vi "Get Profile Extract Cnt.vi"(8 "Profile Cnt (0: rest)":u32, 9 "Profile Index (0)":u32, 10 "Profile Info":T1, 11 "Profile Data":u32[](array[numeric])) -> (3 "Extract Cnt":u32)   [LabVIEW 2014, in "Keyence LJ-V7000.lvlib"]
uses:
  Keyence LJ-V7000.lvlib
  Public/Clusters/Profile Info.ctl
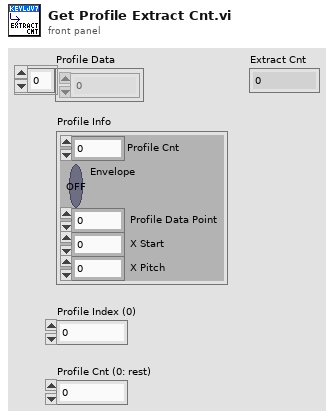
[diagram p1: front panel]
types:
  T1 = typedef "Keyence LJ-V7000.lvlib/Profile Info.ctl" = cluster{"Profile Cnt":u8, "Envelope":bool, " Profile Data Point":u16, " X Start":i32, " X Pitch":i32}
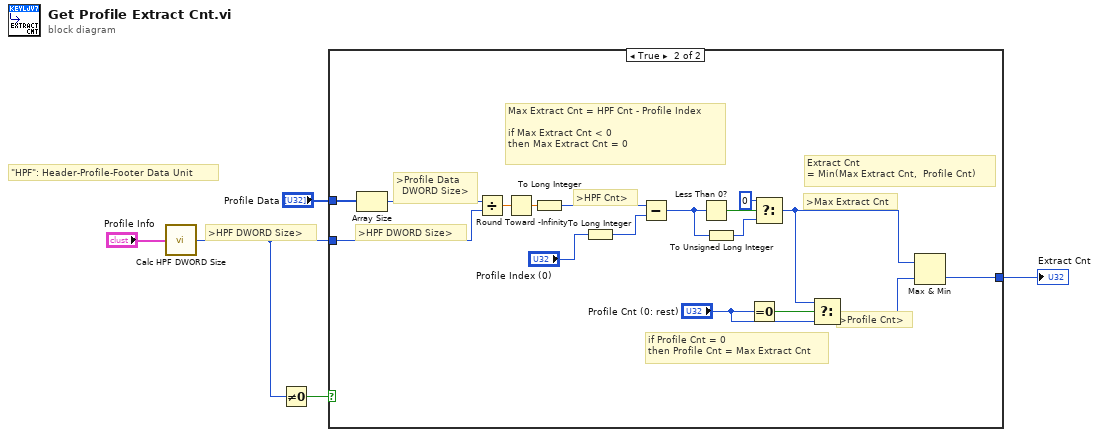
[diagram p0: block diagram]
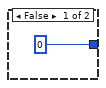
[diagram p2: hidden frame]
diagram:
  # ">HPF DWORD Size>"
  # "\"HPF\": Header-Profile-Footer Data Unit"
  n1 = call "Calc HPF DWORD Size.vi"("Profile Info"="Profile Info") -> ("DWORD Size"=w1:u32)  [unwired: 4 in]
  n2 = Not Equal To 0?(x=w1) -> (x != 0?=w2:bool)
  n3 = case shown="True" w2 {
    tunnel: "Profile Data" -> [_ w23]
    tunnel: [u32 0 w22] -> w3
    tunnel: w1 -> [_ w20]
    frame False {
    }
    frame True {
      # ">HPF DWORD Size>"
      # ">HPF Cnt>"
      # ">Profile Data \n  DWORD Size>"
      # ">Max Extract Cnt"
      # ">Profile Cnt>"
      # "Extract Cnt\n= Min(Max Extract Cnt,  Profile Cnt)"
      # "if Profile Cnt = 0\nthen Profile Cnt = Max Extract Cnt"
      # "Max Extract Cnt = HPF Cnt - Profile Index\n\nif Max Extract Cnt < 0\nthen Max Extract Cnt = 0"
      n4 = Array Size(array=w23) -> (size(s)=w10:i32)
      n5 = Divide(x=w10, y=w20) -> (x/y=w11:dbl)
      n6 = Round Toward -Infinity(1:w11) -> (0:w12:dbl)
      n7 = To Long Integer(number=w12) -> (32bit integer=w13:i32)
      n8 = To Long Integer(number="Profile Index (0)") -> (32bit integer=w14:i32)
      n9 = Subtract(x=w13, y=w14) -> (x-y=w19:i32)
      n10 = Less Than 0?(x=w19) -> (x < 0?=w16:bool)
      n11 = To Unsigned Long Integer(number=w19) -> (unsigned 32bit integer=w18:u32)
      n12 = Equal To 0?(x="Profile Cnt (0: rest)") -> (x = 0?=w15:bool)
      n13 = Select(t=u32 0, s=w16, f=w18) -> (s? t:f=w8:u32)
      n14 = Select(t=w8, s=w15, f="Profile Cnt (0: rest)") -> (s? t:f=w7:u32)
      n15 = Max & Min(x=w8, y=w7) -> (min(x,y)=w22:u32)  [unwired: 1 out]
    }
  }
  "Extract Cnt" <- w3
